vi "Diff Packages.vi"(8 "error in (no error)":errorcluster, 11 "Artifactory.VIPM in":refnum<class "Artifactory.VIPM.lvclass">) -> (0 "error out":errorcluster, 3 "Artifactory.VIPM out":refnum<class "Artifactory.VIPM.lvclass">)   [LabVIEW 2021, in "Artifactory.VIPM.lvclass"]
uses:
  Artifactory.VIPM.lvclass
  C:/Repositories/LVOS/Artifactory/lv-src/Artifactory/Artifactory.lvclass
  Artifactory/Artifactory.lvclass/Artifactory.ctl
  Artifactory.VIPM.lvclass/Artifactory.VIPM.ctl
  Artifactory/Artifactory.lvclass
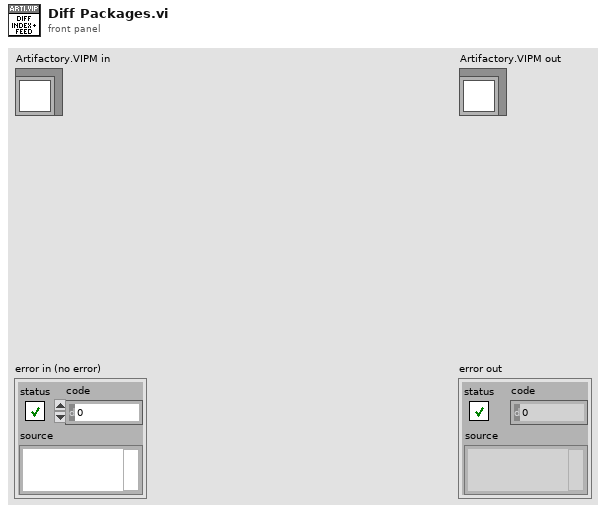
[diagram p1: front panel]
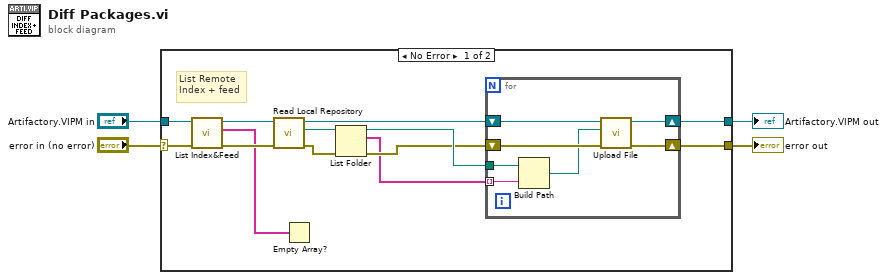
[diagram p0: block diagram]
diagram:
  n1 = case shown="No Error" "error in (no error)" {
    selector: "error in (no error)" -> [w14 w25]
    tunnel: [w13 w25] -> w3
    tunnel: [w16 w24] -> w1
    tunnel: "Artifactory.VIPM in" -> [w15 w24]
    frame No Error {
      # "List Remote\nIndex + feed"
      n2 = call "List Index&Feed.vi"("error in (no error)"=w14, "Artifactory.VIPM in"=w15) -> ("error out"=w8:errorcluster, "Index & Feed"=w6:string[], "Artifactory.VIPM out"=w12:refnum<class "Artifactory.VIPM.lvclass">)  [unwired: 7 in]
      n3 = call "Read Local Repository.vi"("Artifactory in"=w12) -> ("Local Repository"=w10:path, "Artifactory out"=w11:refnum<class "Artifactory.VIPM.lvclass">)  [unwired: 9 in]
      n4 = Empty Array?(array=w6) -> ()  [unwired: 1 out]
      n5 = List Folder(path=w10, error in=w8) -> (path out=w9:path, filenames=w5:string[], error out=w7:errorcluster)  [unwired: 2 in, 1 out]
      n6 = for {
        shift-right: [w22] -> w16
        shift-left: w11 -> [w23]
        shift-right: [w20] -> w13
        shift-left: w7 -> [w21]
        tunnel: w5 -> [w19] mode=indexing
        tunnel: w9 -> [w17]
        n7 = Build Path(base path=w17, name or relative path=w19) -> (appended path=w18:path)
        n8 = call "Upload File.vi"("error in (no error)"=w21, "Local File"=w18, "Artifactory in"=w23) -> ("error out"=w20:errorcluster, "Artifactory out"=w22:refnum<class "Artifactory.VIPM.lvclass">)  [unwired: 7 in]
      }
    }
    frame Error {
    }
  }
  "error out" <- w3
  "Artifactory.VIPM out" <- w1
